vi "Get Session Path.vi"(8 "error in (no error)":errorcluster, 11 "AcquistionObject in":refnum<class "AcquistionObject.lvclass">) -> (0 "error out":errorcluster, 2 "Path":path, 3 "AcquistionObject out":refnum<class "AcquistionObject.lvclass">)   [LabVIEW 2014, in "AcquisitionCoreObjects.lvlib" / "AcquistionObject.lvclass"]
uses:
  AcquistionObject.lvclass
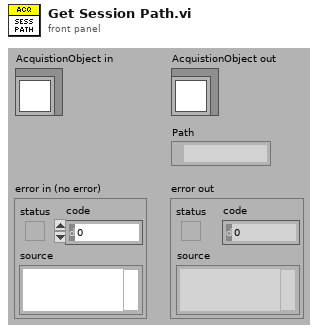
[diagram p1: front panel]
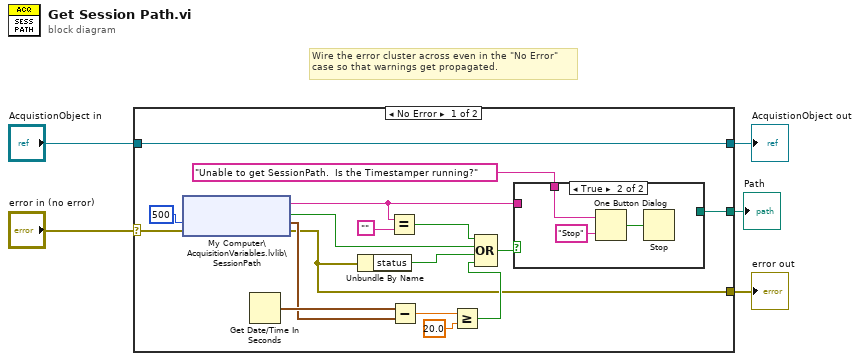
[diagram p0: block diagram]
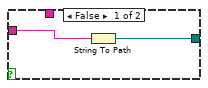
[diagram p2: hidden frame]
diagram:
  # "Wire the error cluster across even in the \"No Error\"\ncase so that warnings get propagated."
  n1 = case shown="No Error" "error in (no error)" {
    selector: "error in (no error)" -> [w7 w29]
    tunnel: [w8 w29] -> w4
    tunnel: [w22 w28] -> w2
    tunnel: "AcquistionObject in" -> [w22 w28]
    tunnel: [w9 _] -> w1
    frame No Error {
      n2 = shared-variable "My Computer\\AcquisitionVariables.lvlib\\SessionPath"(error in=w7, 500 ("ms timeout (0)")) -> (w14:string, error out=w8:errorcluster, w18:bool, w12:timestamp)
      n3 = Get Date/Time In Seconds() -> (seconds since 1Jan1904=w13:timestamp)
      n4 = Unbundle By Name(w8) -> ("status"=w17:bool)
      n5 = Equal?(x=w14, y="") -> (x = y?=w19:bool)
      n6 = Subtract(x=w13, y=w12) -> (x-y=w11:dbl)
      n7 = Greater Or Equal?(x=w11, y=20.0) -> (x >= y?=w10:bool)
      n8 = Compound Arithmetic op=OR(w19, w18, w17, w10) -> (w16:bool)
      n9 = case shown="True" w16 {
        tunnel: "Unable to get SessionPath.  Is the Timestamper running?" ("message") -> [_ w27]
        tunnel: w14 -> [w24 _]
        tunnel: [w23 _] -> w9
        frame False {
          n10 = String To Path(string=w24) -> (path=w23:path)
        }
        frame True {
          n11 = One Button Dialog(message=w27, button name ("OK")="Stop") -> (true=w26:bool)
          n12 = Stop(stop? (T)=w26) -> ()
        }
      }
    }
    frame Error {
    }
  }
  "error out" <- w4
  "AcquistionObject out" <- w2
  "Path" <- w1
